vi "Plugin - Current Time.vi"() -> ()   [LabVIEW 2023]
doc: "Subpanel Plugin VI that displays the current time."
panel:
  out "Current Time":string
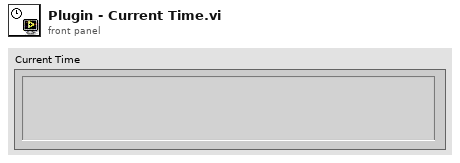
[diagram p1: front panel]
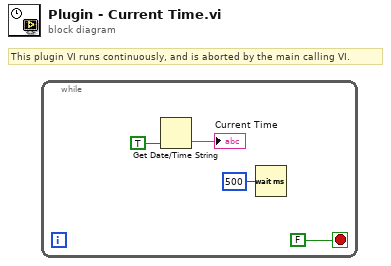
[diagram p0: block diagram]
diagram:
  # "This plugin VI runs continuously, and is aborted by the main calling VI."
  n1 = while {
    stop <- FALSE stop-if-true
    n2 = Get Date/Time String(want seconds? (F)=TRUE) -> (time string=→"Current Time":string)  [unwired: 2 in, 1 out]
    n3 = Wait (ms)(milliseconds to wait=u32 500) -> ()  [unwired: 1 out]
  }
